vi "Read Boolean.vi"(8 "error in (no error)":errorcluster, 11 "Section 1 in":refnum<class "Section 1.lvclass">) -> (0 "error out":errorcluster, 2 "Boolean":bool=TRUE, 3 "Section 1 out":refnum<class "Section 1.lvclass">)   [LabVIEW 2012, in "LVOOP Introduction.lvlib" / "Section 1.lvclass"]
uses:
  Section 1.lvclass
  Section 1.lvclass/Section 1.ctl
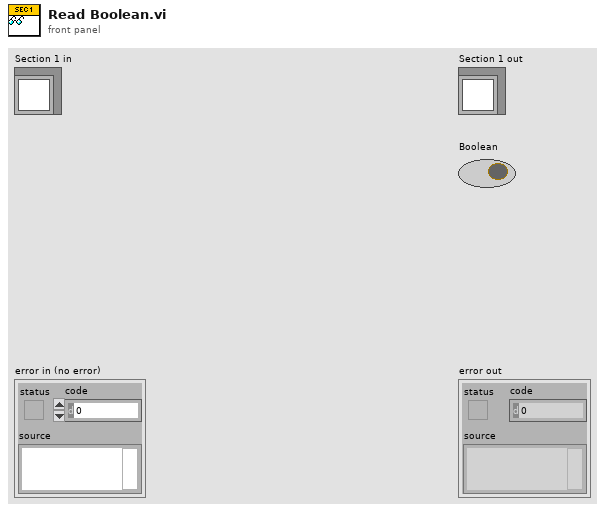
[diagram p1: front panel]
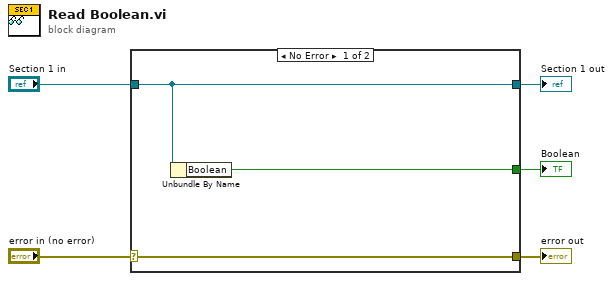
[diagram p0: block diagram]
diagram:
  n1 = case shown="No Error" "error in (no error)" {
    selector: "error in (no error)" -> [w8 w9]
    tunnel: [w8 w9] -> w4
    tunnel: [w7 w10] -> w2
    tunnel: "Section 1 in" -> [w7 w10]
    tunnel: [w6 _] -> w1
    frame No Error {
      n2 = Unbundle By Name(w7) -> ("Boolean"=w6:bool)
    }
    frame Error {
    }
  }
  "error out" <- w4
  "Section 1 out" <- w2
  "Boolean" <- w1
